vi "string log (SubVI).vi"(8 "error in (no error)":errorcluster, 10 "Enum":enum16{"Init", "Log", "Read", "Clear"}(ring)=enum."Log", 11 "state Name":string) -> (0 "error out":errorcluster, 3 "State log":string)   [LabVIEW 2018, in "Application.lvlib"]
uses:
  Application.lvlib
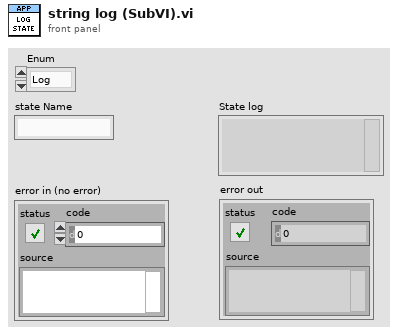
[diagram p1: front panel]
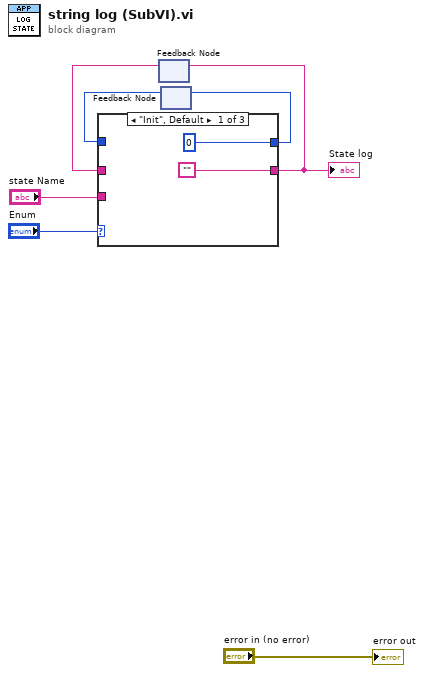
[diagram p0: block diagram]
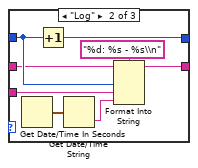
[diagram p2: hidden frame]
diagram:
  n1 = feedback #1() -> (w4:string)  [unwired: 1 in]
  n2 = feedback #2() -> (w6:i32)  [unwired: 1 in]
  n3 = case shown="\"Init\", Default" "Enum" {
    tunnel: "state Name" -> [_ w17 _]
    tunnel: w6 -> [_ w16 w18]
    tunnel: [0 w15 w18] -> w5
    tunnel: w4 -> [_ w13 w19]
    tunnel: ["" w12 w19] -> w1
    frame "Init", Default {
    }
    frame "Log" {
      n4 = Get Date/Time In Seconds() -> (seconds since 1Jan1904=w10:timestamp)
      n5 = Increment(x=w16) -> (x+1=w15:i32)
      n6 = Get Date/Time String(seconds (now)=w10) -> (time string=w11:string)  [unwired: 2 in, 1 out]
      n7 = Format Into String(format string="%d: %s - %s\\n", initial string=w13, w16, w17, w11) -> (resulting string=w12:string)  [unwired: 1 in, 1 out]
    }
    frame "Read" {
    }
  }
  "State log" <- w1
  n8 = feedback-in #1(w1) -> ()
  n9 = feedback-in #2(w5) -> ()
  "error out" <- "error in (no error)"
